vi "Simulation Time Advance.vi"(8 "error in (no error)":errorcluster, 11 "simulator":T6={"configuration"={"maxTime"=5.0, "enableVisualization"=TRUE, "Environment Definition"=path "irobotNavigationStateMachine.vi", "Record Location"=path "Simulation Record.xml", "autograde?"=TRUE, "interactive?"=FALSE, "Feedback Mode"=enum."debug navigation", "Robot State Charts"=[path "C:/Users/blueuser/Desktop/Robo Sim Berkley/cpsgrader-release-0.4/Simulators/EECS149lab/src/LabVIEW/statechart/Simulation Statechart.vi"], "statechart"=path "C:/Users/blueuser/Desktop/Robo Sim Berkley/cpsgrader-release-0.4/Simulators/EECS149lab/src/LabVIEW/statechart/Simulation Statechart.vi"}, "Statechart\ndisplay"=refnum, "first step?"=FALSE, "Robots Simulation Statecharts"=[], "Robots"=[]}) -> (0 "error out":errorcluster, 2 "Robot Sensors":T1[](array[typedef]) {"Kobuki Sensors"."Charger Source" items=["DISCHARGING"=0, "DOCKING_CHARGED"=2, "DOCKING_CHARGING"=6, "ADAPTER_CHARGED"=18, "ADAPTER_CHARGING"=22]; "accelerometer"."z axis (g)" format="%.3f"; "accelerometer"."y axis (g)" format="%.3f"; "accelerometer"."x axis (g)" format="%.3f"}, 3 "simulator":T6={"configuration"={"maxTime"=5.0, "enableVisualization"=TRUE, "Environment Definition"=path "irobotNavigationStateMachine.vi", "Record Location"=path "Simulation Record.xml", "autograde?"=TRUE, "interactive?"=FALSE, "Feedback Mode"=enum."debug navigation", "Robot State Charts"=[path "C:/Users/blueuser/Desktop/Robo Sim Berkley/cpsgrader-release-0.4/Simulators/EECS149lab/src/LabVIEW/statechart/Simulation Statechart.vi"], "statechart"=path "C:/Users/blueuser/Desktop/Robo Sim Berkley/cpsgrader-release-0.4/Simulators/EECS149lab/src/LabVIEW/statechart/Simulation Statechart.vi"}, "Statechart\ndisplay"=refnum, "first step?"=FALSE, "Robots Simulation Statecharts"=[], "Robots"=[]})   [LabVIEW 2015]
uses:
  Simulator.ctl
  CyberSim interface/Simulation Configuration.ctl
  autograder/feedbackMode.ctl
  Multi Bot Code/RobotData.ctl
  <instrlib>/DC Motor Controller/HAIOL/DC Motor Controller.lvclass
  shared/Sensors.ctl
  shared/Accelerometer.ctl
  Kobuki/KobukiSensors.ctl
  Kobuki/Kobuki Bumps and WheelDrops.ctl
  Kobuki/Kobuki Buttons.ctl
  <vilib>/robotics/Simulator/NI_Robotics_Simulator.lvlib
panel:
  # "Electrical: charging, battery, OI mode"
  # "Sensors: bump, cliff, button, wheel drop"
  # "Motors:"
  # "Inertia"
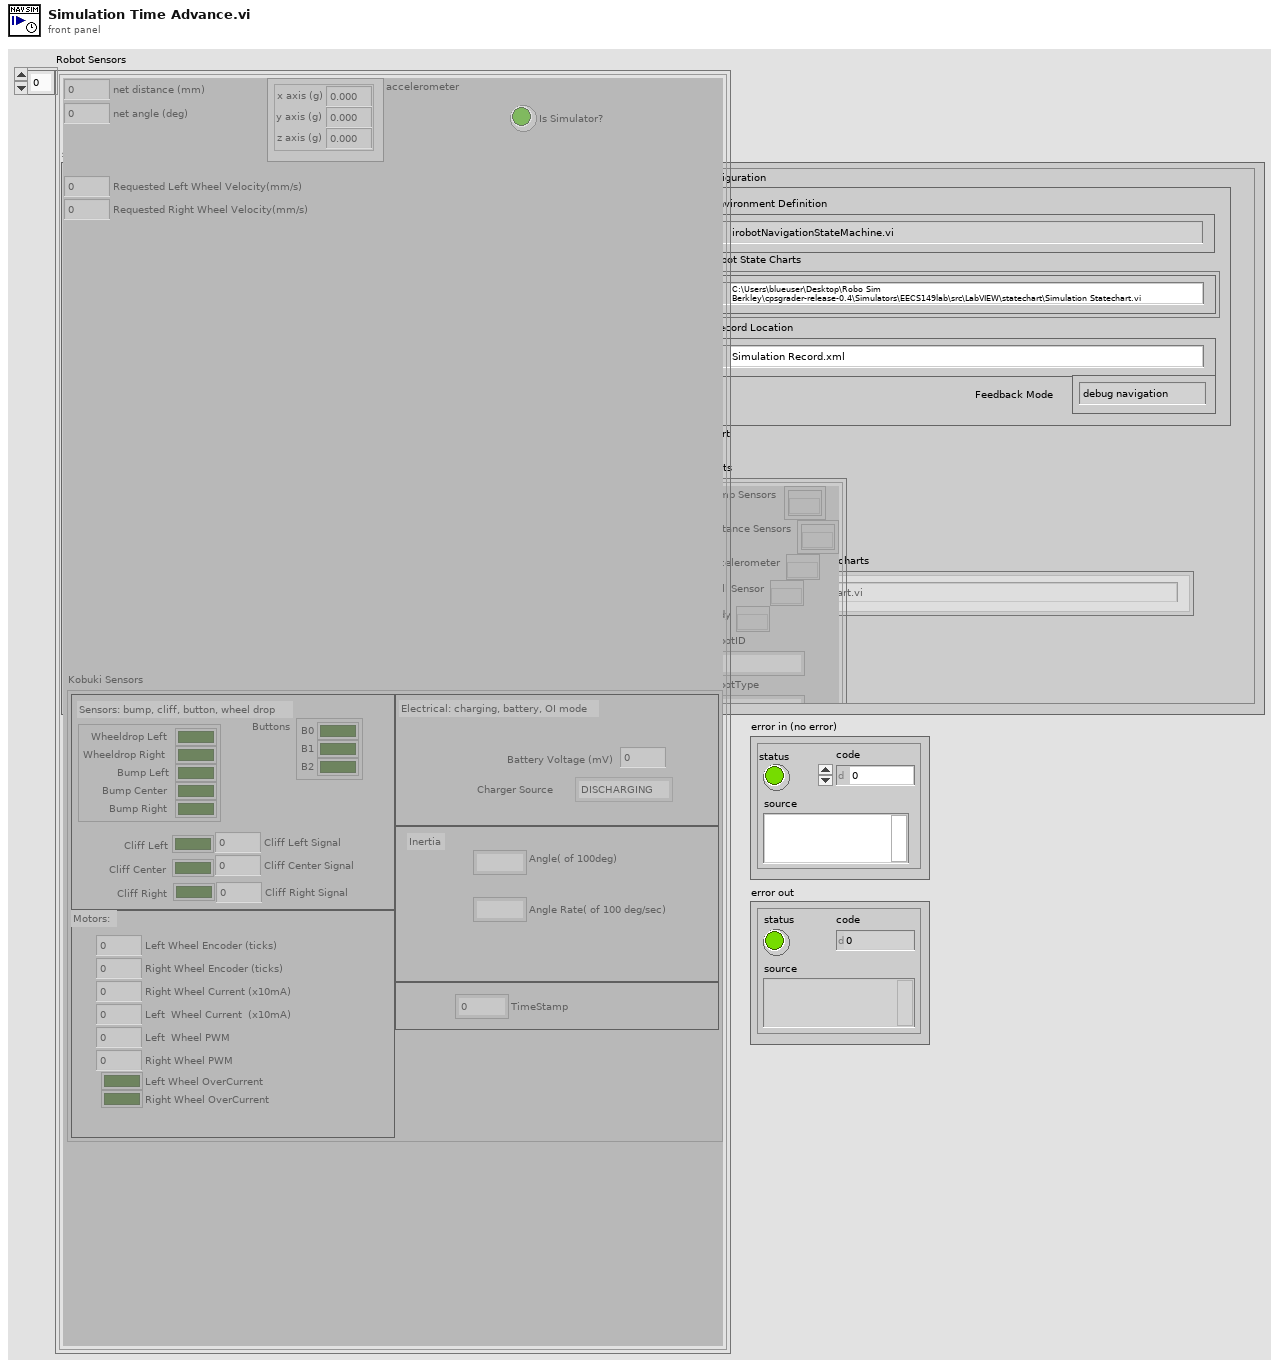
[diagram p1: front panel]
types:
  T1 = typedef "Sensors.ctl" = cluster{"net distance (mm)":i32, "net angle (deg)":i32, "accelerometer":T2, "Is Simulator?":bool, "Kobuki Sensors":T3, "Requested Left Wheel Velocity(mm/s)":i32, "Requested Right Wheel Velocity(mm/s)":i32}
  T2 = typedef "Accelerometer.ctl" = cluster{"x axis (g)":dbl, "y axis (g)":dbl, "z axis (g)":dbl}
  T3 = typedef "KobukiSensors.ctl" = cluster{"Bumps + Wheel Drops":T4, "Cliff Left":bool, "Cliff Center":bool, "Cliff Right":bool, "Cliff Left Signal":u16, "Cliff Center Signal":u16, "Cliff Right Signal":u16, "Buttons":T5, "Left Wheel Encoder (ticks)":u16, "Right Wheel Encoder (ticks) ":u16, "Left  Wheel PWM":i8, "Right Wheel PWM":i8, "Left Wheel OverCurrent":bool, "Right Wheel OverCurrent ":bool, "Right Wheel Current (x10mA)":i16, "Left  Wheel Current  (x10mA)":i16, "TimeStamp":u16, "Battery Voltage (mV)":i16, "Angle( of 100deg)":i16, "Angle Rate( of 100 deg/sec)":i16, "Charger Source ":i8}
  T4 = typedef "Kobuki Bumps and WheelDrops.ctl" = cluster{"Wheeldrop Left":bool, "Wheeldrop Right":bool, "Bump Left":bool, "Bump Center":bool, "Bump Right":bool}
  T5 = typedef "Kobuki Buttons.ctl" = cluster{"B0":bool, "B1":bool, "B2":bool}
  T6 = typedef "Simulator.ctl" = cluster{"configuration":T7, "Statechart\ndisplay":refnum<vi>, "first step?":bool, "Robots Simulation Statecharts":path[], "Robots":T9[]}
  T7 = typedef "Simulation Configuration.ctl" = cluster{"maxTime":sgl, "enableVisualization":bool, "Environment Definition":path, "Record Location":path, "autograde?":bool, "interactive?":bool, "Feedback Mode":T8, "Robot State Charts":path[], "statechart":path}
  T8 = typedef "feedbackMode.ctl" = enum32{"debug navigation", "debug hill climb", "autograde navigation", "autograde hill climb"}
  T9 = typedef "RobotData.ctl" = cluster{"Bump Sensors":refnum<k20>[], "Distance Sensors":refnum<k20>[], "Accelerometer":refnum<k20>, "Wall Sensor":refnum<k20>, "Body":refnum<k20>, "RobotID":string, "RobotType":string, "Left Motor":refnum<class "DC Motor Controller.lvclass">, "Right Motor":refnum<class "DC Motor Controller.lvclass">}
  T10 = typedef "Sim Sensors Feedback.ctl" = cluster{"Position":sgl[], "Position 2":dbl, "yaw":dbl, "net angle":dbl}
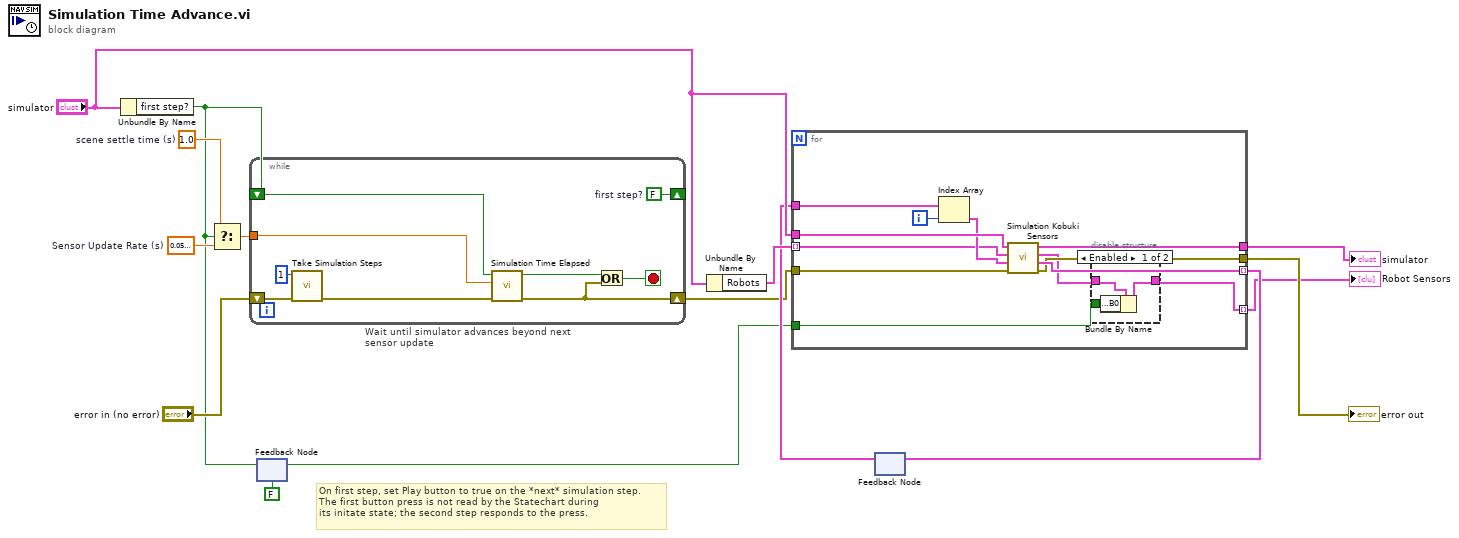
[diagram p0: block diagram]
diagram:
  w14 = sgl 1.0  # scene settle time (s)
  w13 = sgl 0.06  # Sensor Update Rate (s)
  # "On first step, set Play button to true on the *next* simulation step.\nThe first button press is not read by the Statechart during\nits initate state; the second step responds to the press."
  n1 = Unbundle By Name("simulator") -> ("first step?"=w10:bool)
  n2 = Select(t=w14, s=w10, f=w13) -> (s? t:f=w12:sgl)
  n3 = while "Wait until simulator advances beyond next sensor update" {
    shift-right: [w20] -> w5
    shift-left: "error in (no error)" -> [w22]
    shift-right: [w17] -> _
    shift-left: w10 -> [w19]
    tunnel: w12 -> [w18]
    stop <- w21 stop-if-true
    w17 = FALSE  # first step?
    n4 = call <vilib>:"Take Simulation Steps.vi"("error in (no error)"=w22, "number of steps"=u64 1) -> ("error out"=w23:errorcluster)  [unwired: 9 in]
    n5 = call "Simulation Time Elapsed.vi"("error in (no error)"=w23, "Time Target (s)"=w18, "first step?"=w19) -> ("error out"=w20:errorcluster, "Time Elapsed?"=w16:bool)  [unwired: 6 in, 1 out]
    n6 = Or(x=w16, y=w20) -> (x .or. y?=w21:bool)
  }
  n7 = feedback #1(FALSE ("init?")) -> (w4:bool)
  n8 = feedback-in #1(w10) -> ()
  n9 = Unbundle By Name("simulator") -> ("Robots"=w9:T9[])
  n10 = feedback #2() -> (w6:T10[])  [unwired: 1 in]
  n11 = for {
    tunnel: w9 -> [w28] mode=indexing
    tunnel: "simulator" -> [w36]
    tunnel: [w35] -> w3
    tunnel: [w34] -> w7 mode=indexing
    tunnel: [w33] -> w2
    tunnel: w6 -> [w30]
    tunnel: w5 -> [w32]
    tunnel: w4 -> [w26]
    tunnel: [w27] -> w1 mode=indexing
    i -> [w31]
    n12 = Index Array(array=w30, index=w31) -> (element=w29:T10)
    n13 = call "Simulation Kobuki Sensors.vi"("error in"=w32, "Feedback Input"=w29, "Robot"=w28, "simulator"=w36) -> ("error out"=w33:errorcluster, "Feedback Output"=w34:T10, "sensors"=w25:T1, "simulator"=w35:T6)  [unwired: 4 in]
    n14 = disable-structure shown="Enabled" {
      disable-tunnel: [w39 w40] -> w27
      disable-tunnel: w26 -> [w38 _]
      disable-tunnel: w25 -> [w37 w40]
      frame Enabled {
        n15 = Bundle By Name(cluster=w37, "Kobuki Sensors.Buttons.B0"=w38) -> (w39:T1)
      }
      frame Disabled {
      }
    }
  }
  "simulator" <- w3
  "error out" <- w2
  "Robot Sensors" <- w1
  n16 = feedback-in #2(w7) -> ()
